vi "TSPopup.Tree Show Popup.vi"(0 "Numeric":i64, 3 "String":string) -> (5 "Prop Type":T1)   [LabVIEW 2016, in "TSPopup.lvlib" / "TSPopup.lvclass"]
doc: "Invokes the Type Sensitive Popup using the provided Parameters. This <B>MUST</B> be used in the 'Mouse Down<B>?</B>' event, which is the filtering event. This makes the popup visible before allowing the mouse click to be handled.\n\n<B>Popup Parameters</B> - Parameters for showing the Type Sensitive Popup.\n<B>Call data</B> - This input will be returned with the 'Popup Event' for use in handling the Popup results.\n<B>Font Size</B> - If wired, this sets the font size of popups.\n\nType Sensitive Popup \nCopyright © 2007, J. David Saunders\nAll rights reserved."
uses:
  <userlib>/TSPopup/TSPopup.lvclass
  <userlib>/TSPopup/TSPopup.Data Type.ctl
panel:
  # "Type Sensitive Popup \nCopyright © 2007, J. David Saunders\nAll rights reserved."
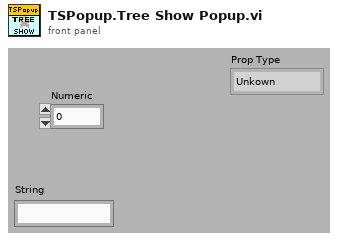
[diagram p1: front panel]
types:
  T1 = typedef "TSPopup.lvlib/TSPopup.lvclass/TSPopup.Data Type.ctl" = enum16{"Unkown", "NO POPUP", "String", "Integer", "Float", "Color", "Boolean", "Ring", "Captioned String", "Captioned Integer", "Button Color", "2 Int Cluster", "4 Int Cluster", "check"}
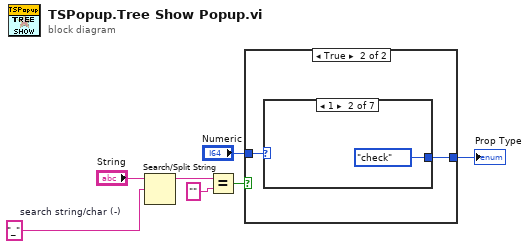
[diagram p0: block diagram]
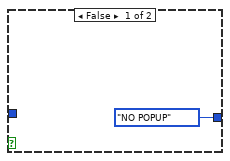
[diagram p2: hidden frame]
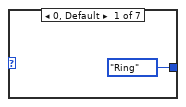
[diagram p3: hidden frame]
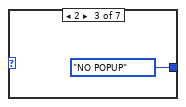
[diagram p4: hidden frame]
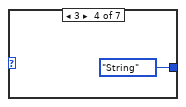
[diagram p5: hidden frame]
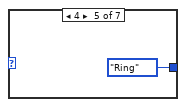
[diagram p6: hidden frame]
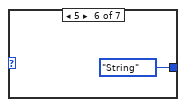
[diagram p7: hidden frame]
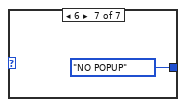
[diagram p8: hidden frame]
diagram:
  w5 = "_"  # search string/char (-)
  n1 = Search/Split String(string="String", search string/char (-)=w5) -> (substring before match=w3:string)  [unwired: 1 in, 2 out]
  n2 = Equal?(x=w3, y="") -> (x = y?=w1:bool)
  n3 = case shown="True" w1 {
    tunnel: "Numeric" -> [_ w10]
    tunnel: [TSPopup.Data_Type."NO POPUP" ("Prop Type") w9] -> w6
    frame False {
    }
    frame True {
      n4 = case shown="1" w10 {
        tunnel: [TSPopup.Data_Type."Ring" ("Prop Type") TSPopup.Data_Type."check" ("Prop Type") TSPopup.Data_Type."NO POPUP" ("Prop Type") TSPopup.Data_Type."String" ("Prop Type") TSPopup.Data_Type."Ring" ("Prop Type") TSPopup.Data_Type."String" ("Prop Type") TSPopup.Data_Type."NO POPUP" ("Prop Type")] -> w9
        frame 0, Default {
        }
        frame 1 {
        }
        frame 2 {
        }
        frame 3 {
        }
        frame 4 {
        }
        frame 5 {
        }
        frame 6 {
        }
      }
    }
  }
  "Prop Type" <- w6
